vi "PH_Countdown-Counter.ProcEvents.vi"(0 "i ref in":refnum<vi>, 5 "error in (no error)":errorcluster) -> (14 "i ref out":refnum<vi>, 19 "error out":errorcluster)   [LabVIEW 2014, in "PH_Countdown-Counter.lvlib"]
doc: "This method is used to define the events the object will listen to. Add your own events here."
uses:
  PH_Countdown-Counter.lvlib
  CS_Core/BaseProcess/BaseProcess.lvlib
  PH_Basics/PH_Common/PH_Common.lvlib
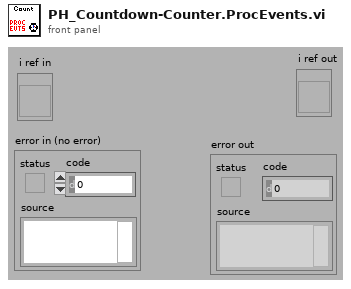
[diagram p1: front panel]
types:
  T1 = typedef "PH_Countdown-Counter.lvlib/PH_Countdown-Counter.i attribute.ctl" = cluster{"Machine Time":cluster{"Tag":string, "Wating Time [s]":dbl, "not linked?":bool}[], "Last Shot":cluster{"Tag":string, "Shot Time [s]":timestamp, "not linked?":bool}[], "Time since last Shot?":bool, "Calculation":cluster{"Time between Shots [s]":dbl, "Ref Remaining Time":refnum<vi>, "Service ID":i32, "over?":bool, "Ref Time between Shots":refnum<vi>, "Ref Set Mode":refnum<vi>}, "Sound?":bool, "Reminder":cluster{"# 1":cluster{"Pretime [s]":dbl, "Aktive?":bool, "Over?":bool}, "# 2":cluster{"Pretime [s]":dbl, "Aktive?":bool, "Over?":bool}}, "MainAmp only":cluster{"State":bool, "GUI Ref":refnum<vi>}}
  T2 = cluster{"Tag":string, "Wating Time [s]":dbl, "not linked?":bool}[]
  T3 = cluster{"Tag":string, "Shot Time [s]":timestamp, "not linked?":bool}[]
  T4 = typedef "PH_Common.lvlib/PH_DIM.Event Declarer.ctl" = cluster{"Service Name":string, "Selector":string}
  T5 = typedef "BaseProcess.lvlib/BaseProcess.event definition.ctl" = cluster{"CAEEvtDef":T6, "Data Descriptor":T7}
  T6 = typedef "CAEObj.lvlib/CAEObj.event definition.ctl" = cluster{"URL":string, "enable":bool, "ignoreResID":bool}
  T7 = typedef "BaseProcess.lvlib/BaseProcess.descriptor string definition.ctl" = string
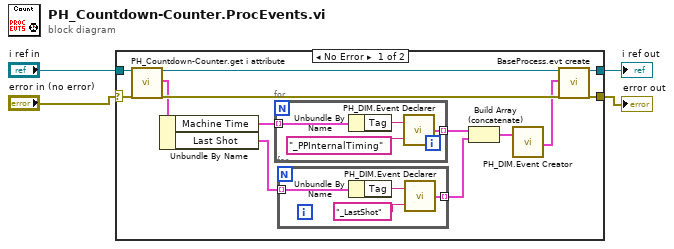
[diagram p0: block diagram]
diagram:
  n1 = case shown="No Error" "error in (no error)" {
    selector: "error in (no error)" -> [w12 w26]
    tunnel: "i ref in" -> [w15 w27]
    tunnel: [w14 w27] -> w3
    tunnel: [w13 w26] -> w2
    frame No Error {
      n2 = call "PH_Countdown-Counter.get i attribute.vi"("i ref in"=w15, "error in (no error)"=w12) -> ("i ref out"=w17:refnum<vi>, "i attribute"=w10:T1, "error out"=w16:errorcluster)  [unwired: 15 in]
      n3 = Unbundle By Name(w10) -> ("Machine Time"=w7:T2, "Last Shot"=w6:T3)
      n4 = for {
        tunnel: [w24] -> w9 mode=indexing
        tunnel: w7 -> [w23] mode=indexing
        n5 = Unbundle By Name(w23) -> ("Tag"=w22:string)
        n6 = call "PH_DIM.Event Declarer.vi"("Selector"="_PPInternalTiming" ("URL"), "Service Name"=w22) -> ("declared DIM Event"=w24:T4)
      }
      n7 = for {
        tunnel: [w20] -> w5 mode=indexing
        tunnel: w6 -> [w19] mode=indexing
        n8 = Unbundle By Name(w19) -> ("Tag"=w18:string)
        n9 = call "PH_DIM.Event Declarer.vi"("Selector"="_LastShot" ("URL"), "Service Name"=w18) -> ("declared DIM Event"=w20:T4)
      }
      n10 = Build Array (concatenate)(w9, w5) -> (w11:T4[])
      n11 = call "PH_DIM.Event Creator.vi"("Trendmessage Services"=w11) -> ("DIM Service Events"=w8:T5[])  [unwired: 18 in]
      n12 = call "BaseProcess.evt create.vi"("i ref in"=w17, "newEvents"=w8, "error in (no error)"=w16) -> ("i ref out"=w14:refnum<vi>, "error out"=w13:errorcluster)  [unwired: 13 in, 2 out]
    }
    frame Error {
    }
  }
  "i ref out" <- w3
  "error out" <- w2
